vi "Gyroscope Correct GPT.vi"(2 "Check":dbl, 4 "YAW":dbl) -> (0 "Out motor":dbl, 1 "Ok":bool)   [LabVIEW 2020]
uses:
  <vilib>/Platform/TimedLoop/XDataNode/timing_clust.ctl
  <vilib>/Platform/TimedLoop/XDataNode/nitl_modes.ctl
  <vilib>/Platform/TimedLoop/XDataNode/wakeup.ctl
  <vilib>/Platform/TimedLoop/XDataNode/XDataNode.xnode
  <vilib>/Platform/TimedLoop/XDataNode/XDNodeRunTimeDep.lvlib
panel:
  out "coerced(x)":dbl
  out "check - motor":bool
  out "yaw - motor":bool
  out "yaw - check":bool
  out "Rez":dbl
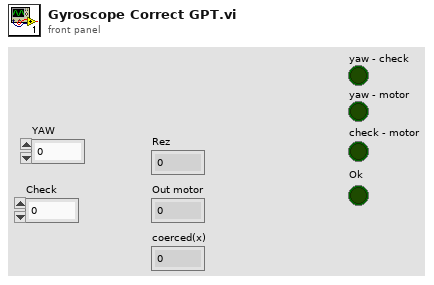
[diagram p1: front panel]
types:
  T1 = typedef "XDNodeRunTimeDep.lvlib/timing_clust.ctl" = cluster{"Expected End [f-1]":u64, "Actual End [f-1]":u64, "Finished Late? [f-1]":bool, "Expected End [i-1]":u64, "Actual End [i-1]":u64, "Finished Late? [i-1]":bool, "Expected Start [i]":u64, "Actual Start [i]":u64, "Expected Start [f]":u64, "Actual Start [f]":u64, "Source Name":string, "Structure Name":string, "Period":i64, "Deadline":i64, "Offset":i64, "Start":i64, "Priority":i32, "Timeout":i32, "Mode":T2, "Wakeup Reason":T3, "Error":errorcluster, "Source Type":string, "Secondary Source Type":string, "Global End Time":u64, "Global Start Time":u64, "Frame Duration":u64, "Iteration Duration":u64, "Assigned CPU":i32, "I/O Scan Engine Mode":u32}
  T2 = typedef "XDNodeRunTimeDep.lvlib/nitl_modes.ctl" = enum32{"No Change", "Process missed periods, maintain original phase", "Discard missed periods, maintain original phase", "Process missed periods, ignore original phase", "Discard missed periods, ignore original phase"}
  T3 = typedef "XDNodeRunTimeDep.lvlib/wakeup.ctl" = enum32{"Normal", "Aborted", "Asynchronous wakeup", "Timing source error", "Timed loop error", "Timeout"}
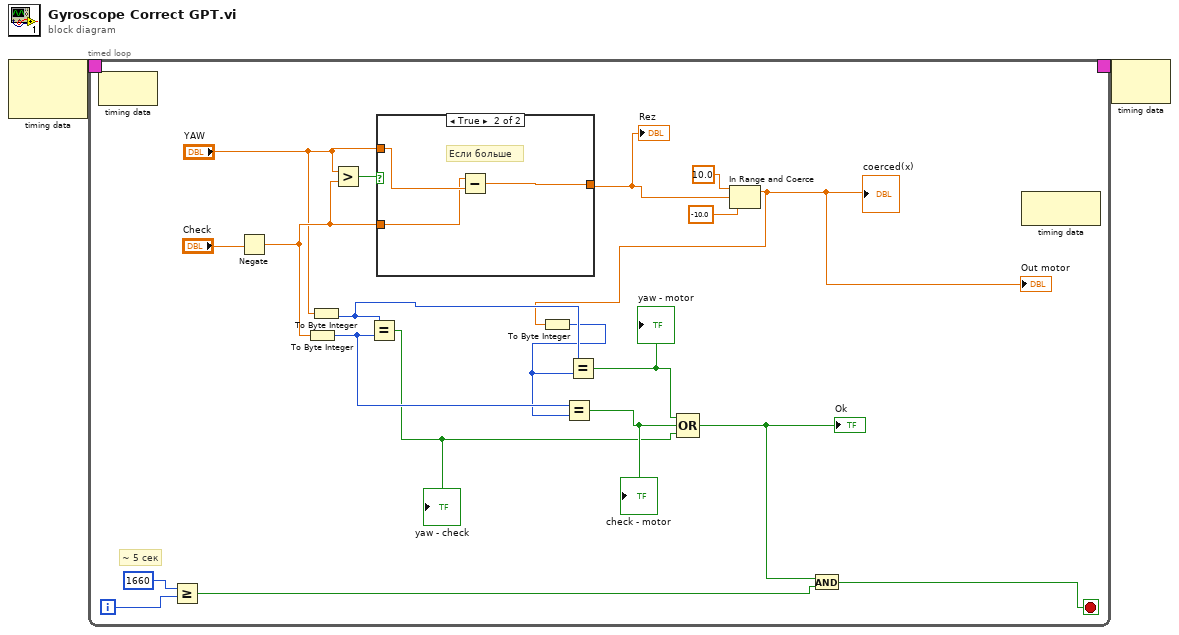
[diagram p0: block diagram]
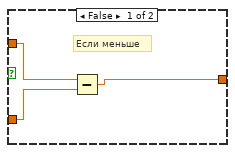
[diagram p2: hidden frame]
diagram:
  n1 = node-c288() -> (w2:T1)  [unwired: 2 in]
  n2 = timed-loop {
    timing: w2 -> [_]
    timing-out: [_] -> w1
    i -> [w7]
    stop <- w3 stop-if-true
    # "~ 5 сек"
    n3 = node-c288() -> ()  [unwired: 1 in, 1 out]
    n4 = Greater Or Equal?(x=1660, y=w7) -> (x >= y?=w4:bool)
    n5 = Negate(x="Check") -> (-x=w12:dbl)
    n6 = To Byte Integer(number=w12) -> (8bit integer=w17:i8)
    n7 = To Byte Integer(number="YAW") -> (8bit integer=w18:i8)
    n8 = Greater?(x="YAW", y=w12) -> (0:w21:bool)
    n9 = Equal?(x=w18, y=w17) -> (x = y?=w11:bool)
    "yaw - check" <- w11
    n10 = case shown="True" w21 {
      tunnel: "YAW" -> [w23 w26]
      tunnel: w12 -> [w22 w25]
      tunnel: [w24 w27] -> w13
      frame False {
        # "Если меньше"
        n11 = Subtract(x=w23, y=w22) -> (x-y=w24:dbl)
      }
      frame True {
        # "Если больше"
        n12 = Subtract(x=w25, y=w26) -> (x-y=w27:dbl)
      }
    }
    "Rez" <- w13
    n13 = In Range and Coerce(upper limit=10.0, x=w13, lower limit=-10.0) -> (coerced(x)=w8:dbl)  [unwired: 1 out]
    "Out motor" <- w8
    "coerced(x)" <- w8
    n14 = To Byte Integer(number=w8) -> (8bit integer=w16:i8)
    n15 = Equal?(x=w17, y=w16) -> (x = y?=w14:bool)
    "check - motor" <- w14
    n16 = Equal?(x=w18, y=w16) -> (x = y?=w15:bool)
    "yaw - motor" <- w15
    n17 = Compound Arithmetic op=OR(w15, w14, w11) -> (w5:bool)
    "Ok" <- w5
    n18 = And(x=w5, y=w4) -> (x .and. y?=w3:bool)
    n19 = node-c288() -> ()  [unwired: 1 in, 1 out]
  }
  n20 = node-c288(w1) -> ()  [unwired: 1 out]
